vi "Close Form.vi"(7 "Name":string, 8 "error in (no error)":errorcluster, 11 "Form Server Wrapper in":refnum<class "Form Server Wrapper.lvclass">) -> (0 "error out":errorcluster, 3 "Form Server Wrapper out":refnum<class "Form Server Wrapper.lvclass">)   [LabVIEW 2020, in "Form Server.lvlib" / "Form Server Wrapper.lvclass"]
uses:
  Form Server Wrapper.lvclass
  Form Server Wrapper.lvclass/Form Server Wrapper.ctl
  Form Server Messages Messages/Close Form Msg/Close Form Msg.lvclass/Close Form Msg.ctl
  <vilib>/ActorFramework/Message Enqueuer/Message Enqueuer.lvclass/Message Enqueuer.ctl
  <vilib>/ActorFramework/Message Enqueuer/Enqueue.vi
  Form Server Messages Messages/Close Form Msg/Close Form Msg.lvclass
  C:/Program Files (x86)/National Instruments/LabVIEW 2020/vi.lib/ActorFramework/Message/Message.lvclass
  <vilib>/ActorFramework/Message Priority Queue/Priority Enqueue.vi
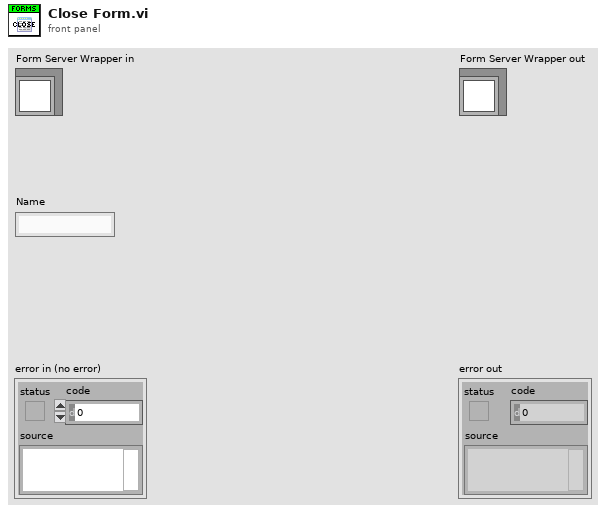
[diagram p1: front panel]
types:
  T1 = typedef "Form Server Interfaces.lvlib/Form ID.ctl" = cluster{"Name":string, "Panel type":string}
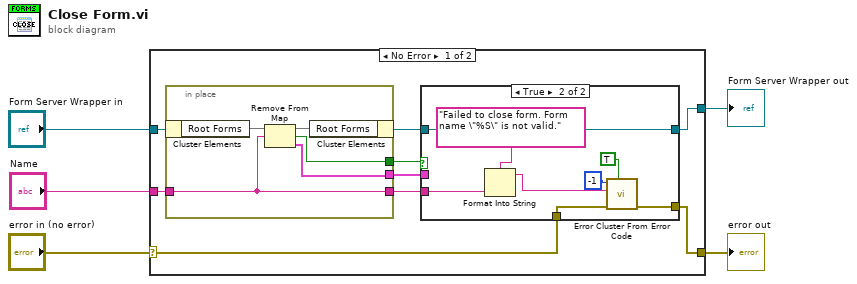
[diagram p0: block diagram]
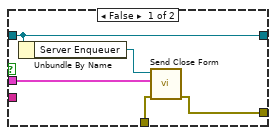
[diagram p2: hidden frame]
diagram:
  n1 = case shown="No Error" "error in (no error)" {
    selector: "error in (no error)" -> [w8 w34]
    tunnel: [w6 w34] -> w4
    tunnel: [w9 w33] -> w2
    tunnel: "Form Server Wrapper in" -> [w14 w33]
    tunnel: "Name" -> [w13 _]
    frame No Error {
      n2 = in-place {
        in-place-border: w13 -> [w28]
        in-place-border: [w30] -> w11
        in-place-border: [w29] -> w12
        in-place-border: [w28] -> w7
        n3 = in-place-cluster #1(w14) -> ("Root Forms"=w32:map{string, T1})
        n4 = Remove From Map(10:w28, 11:w32) -> (1:w30:T1, 2:w29:bool, 3:w31:map{string, T1})
        n5 = in-place-cluster #1("Root Forms"=w31) -> (w10:refnum<class "Form Server Wrapper.lvclass">)
      }
      n6 = case shown="True" w12 {
        tunnel: w11 -> [w17 _]
        tunnel: w10 -> [w19 w24]
        tunnel: [w19 w24] -> w9
        tunnel: w8 -> [w16 w27]
        tunnel: w7 -> [_ w22]
        tunnel: [w15 w20] -> w6
        frame False {
          n7 = Unbundle By Name(w19) -> ("Server Enqueuer"=w18:refnum<class "Message Enqueuer.lvclass">)
          n8 = call "Send Close Form.vi"("error in (no error)"=w16, "Form Name"=w17, "Message Enqueuer"=w18) -> ("error out"=w15:errorcluster)  [unwired: 7 in, 1 out]
        }
        frame True {
          n9 = Format Into String(format string="Failed to close form. Form name \"%S\" is not valid.", w22) -> (resulting string=w21:string)  [unwired: 2 in, 1 out]
          n10 = call <vilib>:"Error Cluster From Error Code.vi"("show call chain? (False)"=TRUE, "error in (no error)"=w27, "error message (\"\")"=w21, "error code (0)"=-1) -> ("error out"=w20:errorcluster)  [unwired: 5 in]
        }
      }
    }
    frame Error {
    }
  }
  "error out" <- w4
  "Form Server Wrapper out" <- w2
